vi "写入物种名.vi"(8 "error in (no error)":errorcluster caption="错误输入（无错误）", 10 "物种名":string, 11 "Animal输入":refnum<class "Animal.lvclass">) -> (0 "error out":errorcluster caption="错误输出", 3 "Animal输出":refnum<class "Animal.lvclass">)   [LabVIEW 2020, in "Animal.lvclass"]
uses:
  Animal.lvclass
  Animal.lvclass/Animal.ctl
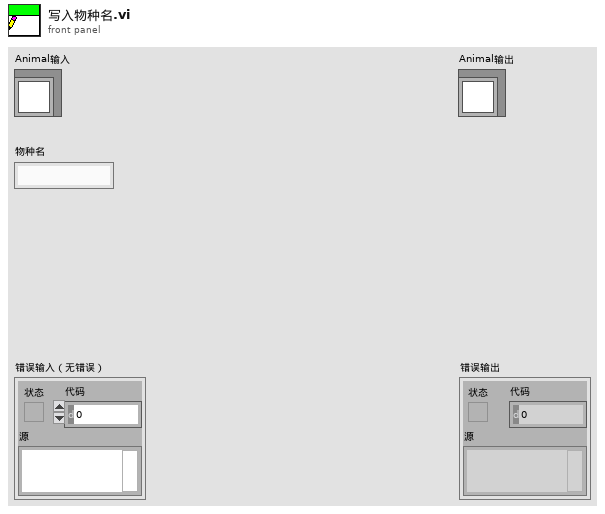
[diagram p1: front panel]
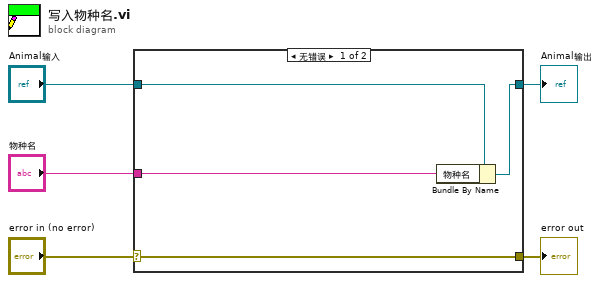
[diagram p0: block diagram]
diagram:
  n1 = case shown="无错误" "error in (no error)" {
    selector: "error in (no error)" -> [w9 w10]
    tunnel: [w9 w10] -> w4
    tunnel: [w7 w11] -> w2
    tunnel: "Animal输入" -> [w8 w11]
    tunnel: "物种名" -> [w6 _]
    frame No Error {
      n2 = Bundle By Name(cluster=w8, "物种名"=w6) -> (w7:refnum<class "Animal.lvclass">)
    }
    frame Error {
    }
  }
  "error out" <- w4
  "Animal输出" <- w2
